vi "Load Profile.vi"(0 "object in":refnum<class "HPS-17000-PowerModule.lvclass">, 5 "profile":dbl[][](array[numeric]), 7 "step dt":i64, 11 "Error In":errorcluster) -> (4 "object out":refnum<class "HPS-17000-PowerModule.lvclass">, 15 "Error Out":errorcluster)   [LabVIEW 2023, in "HPS-17000-PowerModule.lvlib" / "HPS-17000-PowerModule.lvclass"]
uses:
  HPS-17000-PowerModule.lvclass
  <vilib>/HPS-17000/nibatterycycler_grpc_Setpoint.ctl
  <instrlib>/HPS-17000/Internal/Stream Setpoints Multi.vi
  <instrlib>/HPS-17000/HPS-17000.lvclass
  <vilib>/HPS-17000/NI_BC_client.lvlib
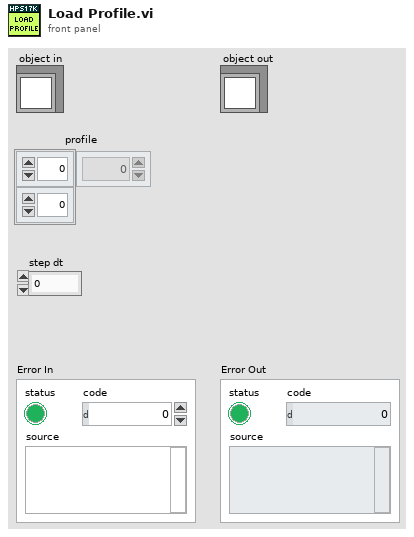
[diagram p1: front panel]
types:
  T1 = typedef "NI_BC_client.lvlib/nibatterycycler_grpc_Setpoint.ctl" = cluster{"voltage":sgl, "current":sgl, "min_power":sgl, "max_power":sgl, "resistance":sgl}
  T2 = typedef "HPS-17000-PowerModule.lvlib/HPS-17000-PowerModule.lvclass/ObjectAttributes.ctl" = cluster{"HPS17000 IP Addresses":string[], "HPS Topology":enum16{"SINGLE", "MULTI"}, "GM ID":string, "TSN NIC IP Address":string, "HPS17000 Refs":refnum<class "HPS-17000.lvclass">[], "Stream Queues":refnum<queue>[], "connected":bool, "reserved":bool, "events":T3, "nibatterycycler_grpc_Setpoint":T1, "last timestamp":i64, "setpoint stream config":T4, "mode":T5, "range":T6}
  T3 = typedef "HPS-17000.lvclass/Multi-Cycler Events.ctl" = cluster{"heartbeats events":refnum<user-event>[], "faults events":refnum<user-event>[], "network sync event":refnum<user-event>[], "setpoint status event":refnum<user-event>[]}
  T4 = typedef "Cycler.lvclass/Setpoint Stream Basic Config.ctl" = cluster{"local address":string, "receiver port":u16}
  T5 = typedef "HPS-17000-PowerModule.lvlib/HPS-17000-PowerModule.lvclass/Mode.ctl" = u16
  T6 = typedef "PowerModuleInterface.lvlibp/PowerModuleInterface.lvclass/Range.ctl" = cluster{"Current Max (A)":dbl, "Current Min (A)":dbl, "Voltage Max (V)":dbl, "Voltage Min (V)":dbl}
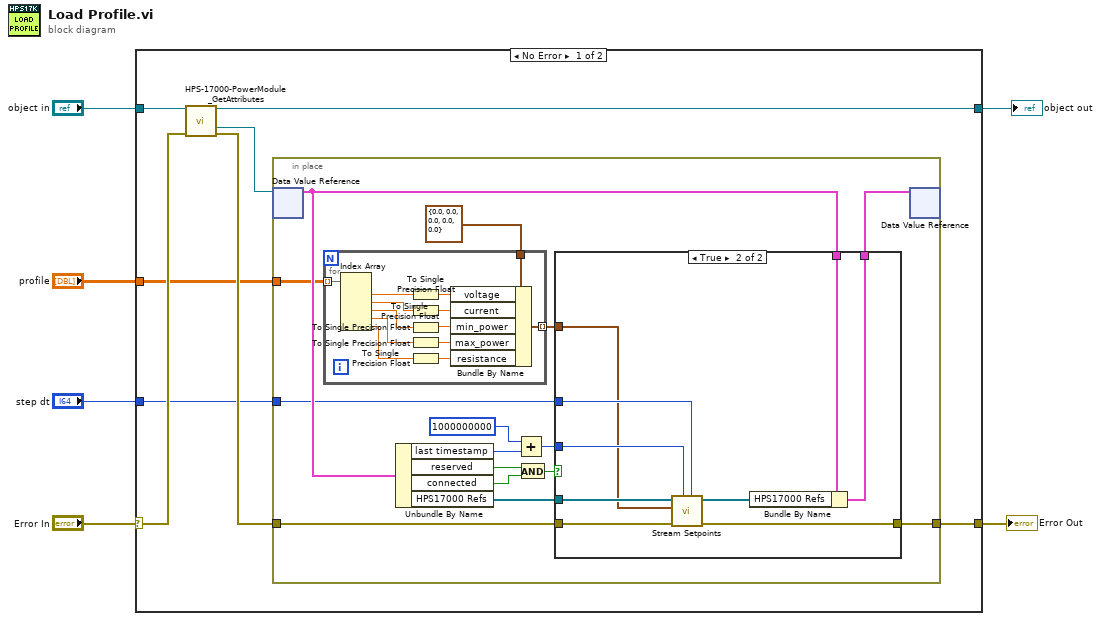
[diagram p0: block diagram]
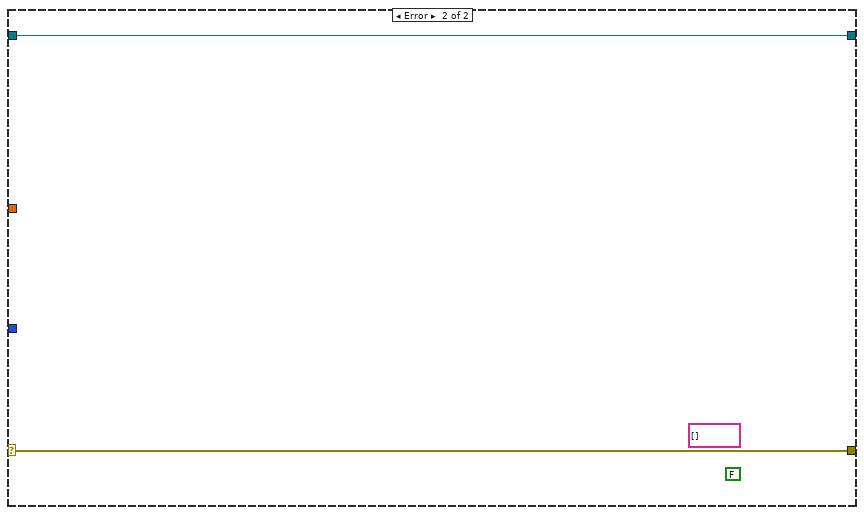
[diagram p3: hidden frame]
diagram:
  n1 = case shown="No Error" "Error In" {
    selector: "Error In" -> [w13 w54]
    tunnel: "object in" -> [w14 w55]
    tunnel: [w9 w55] -> w4
    tunnel: [w10 w54] -> w3
    tunnel: "step dt" -> [w8 _]
    tunnel: "profile" -> [w7 _]
    frame No Error {
      n2 = call "HPS-17000-PowerModule_GetAttributes.vi"("reference in"=w14, "Error In"=w13) -> ("reference out"=w9:refnum<class "HPS-17000-PowerModule.lvclass">, "DataRef"=w12:refnum<data-value>, "Error Out"=w11:errorcluster)  [unwired: 10 in, 1 out]
      n3 = in-place {
        in-place-border: w11 -> [w27]
        in-place-border: [w26] -> w10
        in-place-border: w8 -> [w21]
        in-place-border: w7 -> [w15]
        n4 = in-place-dvr #1(w12) -> (w28:T2)  [unwired: 1 out]
        n5 = for {
          tunnel: T1 {"voltage"=0.0, "current"=0.0, "min_power"=0.0, "max_power"=0.0, "resistance"=0.0} ("nibatterycycler_grpc_Setpoint") -> [w42]
          tunnel: [w41] -> w16 mode=indexing
          tunnel: w15 -> [w40] mode=indexing
          n6 = Index Array(array=w40) -> (element #1=w39:dbl, element #2=w37:dbl, element #3=w36:dbl, element #4=w33:dbl, element #5=w31:dbl)  [unwired: 5 in]
          n7 = To Single Precision Float(number=w39) -> (single precision float=w38:sgl)
          n8 = To Single Precision Float(number=w37) -> (single precision float=w34:sgl)
          n9 = To Single Precision Float(number=w36) -> (single precision float=w35:sgl)
          n10 = To Single Precision Float(number=w33) -> (single precision float=w32:sgl)
          n11 = To Single Precision Float(number=w31) -> (single precision float=w30:sgl)
          n12 = Bundle By Name(cluster=w42, "voltage"=w38, "current"=w34, "min_power"=w35, "max_power"=w32, "resistance"=w30) -> (w41:T1)
        }
        n13 = Unbundle By Name(w28) -> ("last timestamp"=w20:i64, "reserved"=w23:bool, "connected"=w24:bool, "HPS17000 Refs"=w25:refnum<class "HPS-17000.lvclass">[])
        n14 = Add(x=i64 1000000000, y=w20) -> (x+y=w18:i64)
        n15 = And(x=w23, y=w24) -> (x .and. y?=w22:bool)
        n16 = case shown="True" w22 {
          tunnel: [w44 w53] -> w29
          tunnel: w28 -> [w44 w52]
          tunnel: w27 -> [w43 w51]
          tunnel: [w43 w46] -> w26
          tunnel: w25 -> [_ w50]
          tunnel: w21 -> [_ w48]
          tunnel: w18 -> [_ w47]
          tunnel: w16 -> [_ w45]
          frame False {
          }
          frame True {
            n17 = call-poly <instrlib>:"Stream Setpoints.vi"("dt"=w48, "t0"=w47, "error in"=w51, "setpoints"=w45, "cycler refs in"=w50) -> ("error out"=w46:errorcluster, "cycler refs out"=w49:refnum<class "HPS-17000.lvclass">[])  [unwired: 5 in]
            n18 = Bundle By Name(cluster=w52, "HPS17000 Refs"=w49) -> (w53:T2)
          }
        }
        n19 = in-place-dvr #1(w29) -> ()  [unwired: 2 out]
      }
    }
    frame Error {
      (unwired) string[] []
      (unwired) FALSE
    }
  }
  "Error Out" <- w3
  "object out" <- w4
